vi "Shoot_ExecLogic.vi"(9 "Motor2Rpm":dbl, 11 "Motor1Rpm":dbl) -> (3 "CO-ControlOutput":dbl)   [LabVIEW 2025]
uses:
  <vilib>/Rock Robotics/WPI/ThirdParty/JAS_Junk/TrajLib/SlewRateLimiter_New.vi
  <vilib>/Rock Robotics/WPI/ThirdParty/JAS_Junk/TrajLib/SlewRateLimiter_Reset.vi
  <vilib>/Rock Robotics/WPI/ThirdParty/JAS_Junk/TrajLib/SlewRateLimiter_Calculate.vi
  <vilib>/Rock Robotics/WPI/ThirdParty/JAS_Junk/TrajLib/SlewRateLimiter_SetRate.vi
  <vilib>/Rock Robotics/WPI/ThirdParty/JAS_Junk/TrajLib/SimpleMotorFF_Calculate.vi
  <vilib>/Rock Robotics/WPI/ThirdParty/JAS_Junk/TrajLib/VI/Util_GetTime_U32.vi
  <vilib>/Rock Robotics/WPI/ThirdParty/JAS_Junk/TrajLib/PIDController_AtSetpoint.vi
  <vilib>/Rock Robotics/WPI/ThirdParty/JAS_Junk/TrajLib/PIDController_SetPIDF.vi
  <vilib>/Rock Robotics/WPI/ThirdParty/JAS_Junk/TrajLib/PIDController_SetDerivativeFilter.vi
  <vilib>/Rock Robotics/WPI/ThirdParty/JAS_Junk/TrajLib/PIDController_SetIntegratorRange.vi
  <vilib>/Rock Robotics/WPI/ThirdParty/JAS_Junk/TrajLib/PIDController_SetTolerancePandV.vi
  <vilib>/Rock Robotics/WPI/ThirdParty/JAS_Junk/TrajLib/PIDController_DisableContinousInput.vi
  <vilib>/Rock Robotics/WPI/ThirdParty/JAS_Junk/TrajLib/PIDController_EnableContinousInput.vi
  <vilib>/Rock Robotics/WPI/ThirdParty/JAS_Junk/TrajLib/PIDController_Reset.vi
  <vilib>/Rock Robotics/WPI/ThirdParty/JAS_Junk/TrajLib/PIDController_New.vi
  <vilib>/Rock Robotics/WPI/ThirdParty/JAS_Junk/TrajLib/PIDController_SetOutputLimits.vi
  <vilib>/Rock Robotics/WPI/ThirdParty/JAS_Junk/TrajLib/VI/PIDController_SetIntegratorZone.vi
  <vilib>/Rock Robotics/WPI/ThirdParty/JAS_Junk/TrajLib/PIDController_NewPeriod.vi
  <vilib>/Rock Robotics/SystemInterfaces/NetworkCommunication/NetComm_UsageReport_report.vi
  <vilib>/Rock Robotics/SystemInterfaces/Utilities/FPGA_UtilitiesRead LocalTime.vi
  <vilib>/Rock Robotics/WPI/ThirdParty/JAS_Junk/TrajLib/VI/Util_GetTime_U64.vi
  Shoot_Global.vi
  <vilib>/Rock Robotics/Network Tables/NT Write Boolean.vi
  <vilib>/Rock Robotics/Network Tables/NT Write Number.vi
  <vilib>/Rock Robotics/WPI/ThirdParty/JAS_Junk/TrajLib/Globals/Util_LibraryGlobals.vi
  <vilib>/Rock Robotics/WPI/ThirdParty/JAS_Junk/TrajLib/PIDController_AdvCalculate_FF_Sp_Pv.vi
  <vilib>/Rock Robotics/WPI/ThirdParty/JAS_Junk/TrajLib/Trajectory_Library.lvlib
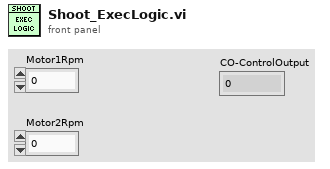
[diagram p1: front panel]
types:
  T1 = typedef "Trajectory_Library.lvlib/SIMPLE_MOTOR_FF.ctl" = cluster{"Ks":dbl, "Kv":dbl, "Ka":dbl, "KnInv":dbl}
  T2 = typedef "Trajectory_Library.lvlib/PID_ADV_LIMITS.ctl" = cluster{"MaxInput":dbl, "MinInput":dbl, "Continuous":bool, "MaxOutput":dbl, "MinOutput":dbl}
  T3 = typedef "Trajectory_Library.lvlib/PID_ADV_TUNING.ctl" = cluster{"Kf":dbl, "Kp":dbl, "Ki":dbl, "Kd":dbl, "MaximumIntegral":dbl, "MinimumIntegral":dbl, "Filter Derivative":bool, "IntegralZone":dbl}
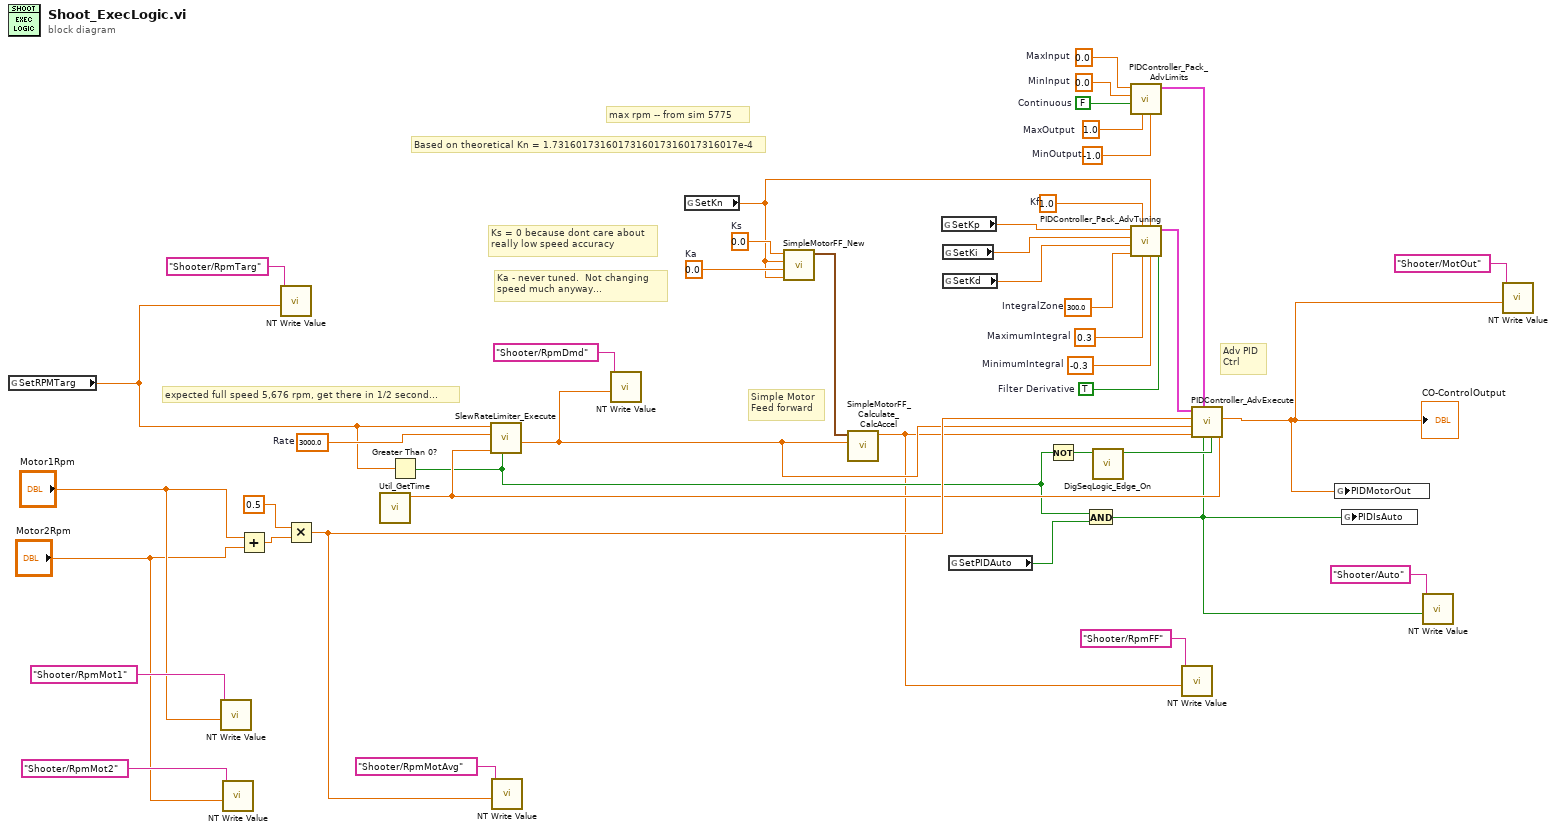
[diagram p0: block diagram]
diagram:
  w32 = 300.0  # IntegralZone
  w31 = 1.0  # Kf
  w30 = 0.3  # MaximumIntegral
  w29 = -0.3  # MinimumIntegral
  w28 = TRUE  # Filter Derivative
  w26 = 0.0  # MinInput
  w25 = FALSE  # Continuous
  w24 = 1.0  # MaxOutput
  w27 = -1.0  # MinOutput
  w23 = 0.0  # MaxInput
  w39 = 0.0  # Ks
  w38 = 0.0  # Ka
  w41 = 3000.0  # Rate
  # "Ka - never tuned.  Not changing\nspeed much anyway..."
  # "Ks = 0 because dont care about\nreally low speed accuracy"
  # "max rpm -- from sim 5775"
  # "Adv PID\nCtrl"
  # "Based on theoretical Kn = 1.7316017316017316017316017316017e-4"
  # "expected full speed 5,676 rpm, get there in 1/2 second..."
  # "Simple Motor\nFeed forward"
  n1 = global read "Shoot_Global.vi" "SetRPMTarg"() -> (w13:dbl)
  n2 = call-poly <vilib>:"NT Write Value.vi"("value"="Motor1Rpm", "name"="Shooter/RpmMot1") -> ()  [unwired: 9 in, 1 out]
  n3 = call-poly <vilib>:"NT Write Value.vi"("value"="Motor2Rpm", "name"="Shooter/RpmMot2") -> ()  [unwired: 9 in, 1 out]
  n4 = Add(x="Motor1Rpm", y="Motor2Rpm") -> (x+y=w35:dbl)
  n5 = call-poly <vilib>:"NT Write Value.vi"("value"=w13, "name"="Shooter/RpmTarg") -> ()  [unwired: 9 in, 1 out]
  n6 = Multiply(x=0.5, y=w35) -> (x*y=w20:dbl)
  n7 = call <vilib>:"Util_GetTime.vi"() -> ("FPGA_Time_Seconds"=w18:dbl)  [unwired: 9 in, 2 out]
  n8 = Greater Than 0?(x=w13) -> (x > 0?=w16:bool)
  n9 = call <vilib>:"SlewRateLimiter_Execute.vi"("Enable"=w16, "Time"=w18, "PositiveRate"=w41, "Input"=w13) -> ("Output"=w19:dbl)  [unwired: 6 in, 1 out]
  n10 = call-poly <vilib>:"NT Write Value.vi"("value"=w20, "name"="Shooter/RpmMotAvg") -> ()  [unwired: 9 in, 1 out]
  n11 = call-poly <vilib>:"NT Write Value.vi"("value"=w19, "name"="Shooter/RpmDmd") -> ()  [unwired: 9 in, 1 out]
  n12 = global read "Shoot_Global.vi" "SetKn"() -> (w4:dbl)
  n13 = call <vilib>:"SimpleMotorFF_New.vi"("Kn"=w4, "Ka"=w38, "Kv"=w4, "Ks"=w39) -> ("SIMPLE_MOTOR_FF"=w40:T1)  [unwired: 7 in]
  n14 = call <vilib>:"SimpleMotorFF_Calculate_CalcAccel.vi"("VelSp"=w19, "SIMPLE_MOTOR_FF"=w40) -> ("FeedForward"=w5:dbl)  [unwired: 9 in]
  n15 = global read "Shoot_Global.vi" "SetKp"() -> (w3:dbl)
  n16 = global read "Shoot_Global.vi" "SetKi"() -> (w2:dbl)
  n17 = global read "Shoot_Global.vi" "SetKd"() -> (w1:dbl)
  n18 = global read "Shoot_Global.vi" "SetPIDAuto"() -> (w14:bool)
  n19 = Not(x=w16) -> (.not. x?=w17:bool)
  n20 = And(x=w16, y=w14) -> (x .and. y?=w7:bool)
  n21 = call <vilib>:"DigSeqLogic_Edge_On.vi"("Input"=w17) -> ("On Edge"=w15:bool)  [unwired: 10 in]
  n22 = call <vilib>:"PIDController_Pack_AdvLimits.vi"("MinOutput"=w27, "MaxOutput"=w24, "Continuous"=w25, "MinInput"=w26, "MaxInput"=w23) -> ("Adv PID Limits"=w21:T2)  [unwired: 6 in]
  n23 = call <vilib>:"PIDController_Pack_AdvTuning.vi"("Filter Derivative"=w28, "MinimumIntegral"=w29, "Kn"=w4, "MaximumIntegral"=w30, "Kf"=w31, "IntegralZone"=w32, "Kd"=w1, "Ki"=w2, "Kp"=w3) -> ("Adv PID Tuning"=w22:T3)  [unwired: 2 in]
  n24 = call-poly <vilib>:"NT Write Value.vi"("value"=w5, "name"="Shooter/RpmFF") -> ()  [unwired: 9 in, 1 out]
  n25 = call <vilib>:"PIDController_AdvExecute.vi"("Time"=w18, "Reset"=w15, "Auto"=w7, "Adv PID Limits"=w21, "FF-FeedForward"=w5, "SP-SetPoint"=w19, "PV-Measurement"=w20, "Adv PID Tuning"=w22) -> ("CO-ControlOutput"=w9:dbl)  [unwired: 1 in, 2 out]
  "CO-ControlOutput" <- w9
  n26 = global write "Shoot_Global.vi" "PIDMotorOut"(w9) -> ()
  n27 = global write "Shoot_Global.vi" "PIDIsAuto"(w7) -> ()
  n28 = call-poly <vilib>:"NT Write Value.vi"("value"=w7, "name"="Shooter/Auto") -> ()  [unwired: 9 in, 1 out]
  n29 = call-poly <vilib>:"NT Write Value.vi"("value"=w9, "name"="Shooter/MotOut") -> ()  [unwired: 9 in, 1 out]
